vi "P2P SPI Master.vi"() -> ()   [LabVIEW 2015]
uses:
  <vilib>/Platform/TimedLoop/XDataNode/timing_clust.ctl
  <vilib>/Platform/TimedLoop/XDataNode/nitl_modes.ctl
  <vilib>/Platform/TimedLoop/XDataNode/wakeup.ctl
  <vilib>/rvi/Emulation/niFpgaSctlEmulationGetInTimedLoop.vi
  <vilib>/rvi/Emulation/niFpgaEmulationReportErrorSimple.vi
  <vilib>/rvi/Emulation/niFpgaGetClockAttributes.vi
  <vilib>/rvi/Emulation/niFpgaCriticalErrorInLSC.vi
  <vilib>/rvi/Emulation/niFpgaEmulationIsFPGAContextNoSignature.vi
  <vilib>/rvi/errors/niFpgaSetErrorForExecOnDevCompSimple.vi
  <vilib>/rvi/eio/common/nirviEmuReportErrorAndStop.vi
  <vilib>/rvi/DataTransferAndStorage/Container/Common/niFpgaContainerGetUniqueNameForEmu.vi
  <vilib>/rvi/FIFO/Fifo_Resource/nirvififoEmulationSetSize.vi
  <vilib>/rvi/FIFO/Fifo_Resource/nirviFifoEmulationQueueMgr.vi
  <instcachedir>/0/nirviFifoEmulationQueueMgr_E5CAEC123FF24DC58D834DCA3CDAA9B5.lvgen/nirviFifoEmulationQueueMgr_E5CAEC123FF24DC58D834DCA3CDAA9B5_001.vi
  <vilib>/Utility/error.llb/Clear Errors.vi
  <vilib>/rvi/FIFO/Fifo_Resource/nirvififoEmulationCreateLock.vi
  <vilib>/rvi/Emulation/niFpgaProcessEmulError.vi
  <vilib>/rvi/FIFO/Fifo_Resource/nirvififoEmulationObtainLock.vi
  <vilib>/rvi/FIFO/Fifo_Resource/nirvififoEmulationReleaseLock.vi
  <vilib>/rvi/occurrence/nirviWaitOnOccurrenceBase.vi
  <vilib>/rvi/errors/nirviReportUnexpectedCaseInternalError.vi
  <vilib>/rvi/errors/nirviReportUnexpectedCaseInternalError (U32).vi
  <vilib>/rvi/eio/common/nirviEmuTemplateMethod_errors.vi
  <vilib>/Platform/TimedLoop/XDataNode/XDataNode.xnode
  <vilib>/rvi/DataTransferAndStorage/Container/XNode/niFpgaContainer.xnode
  <vilib>/rvi/FIFO/Fifo_Resource/nirvififoEmulationRead.vi
  <vilib>/eio/EIONode/EIONode.xnode
  <vilib>/Platform/TimedLoop/XDataNode/XDNodeRunTimeDep.lvlib
  <vilib>/rvi/FIFO/Fifo_Resource/nirvififoEmulationWrite.vi
panel:
  out "SatePassed":u32
  out "clk":bool
  out "t7":bool
  out "t6":bool
  out "t5":bool
  out "t4":bool
  out "t3":bool
  in  "SimSend":bool
  in  "SimData":u32
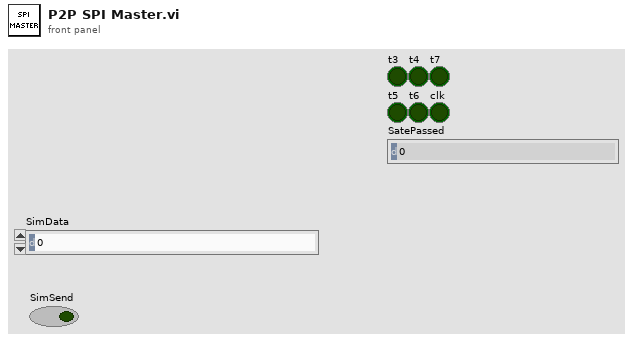
[diagram p1: front panel]
types:
  T1 = typedef "XDNodeRunTimeDep.lvlib/timing_clust.ctl" = cluster{"Expected End [f-1]":u64, "Actual End [f-1]":u64, "Finished Late? [f-1]":bool, "Expected End [i-1]":u64, "Actual End [i-1]":u64, "Finished Late? [i-1]":bool, "Expected Start [i]":u64, "Actual Start [i]":u64, "Expected Start [f]":u64, "Actual Start [f]":u64, "Source Name":string, "Structure Name":string, "Period":i64, "Deadline":i64, "Offset":i64, "Start":i64, "Priority":i32, "Timeout":i32, "Mode":T2, "Wakeup Reason":T3, "Error":errorcluster, "Source Type":string, "Secondary Source Type":string, "Global End Time":u64, "Global Start Time":u64, "Frame Duration":u64, "Iteration Duration":u64, "Assigned CPU":i32, "I/O Scan Engine Mode":u32}
  T2 = typedef "XDNodeRunTimeDep.lvlib/nitl_modes.ctl" = enum32{"No Change", "Process missed periods, maintain original phase", "Discard missed periods, maintain original phase", "Process missed periods, ignore original phase", "Discard missed periods, ignore original phase"}
  T3 = typedef "XDNodeRunTimeDep.lvlib/wakeup.ctl" = enum32{"Normal", "Aborted", "Asynchronous wakeup", "Timing source error", "Timed loop error", "Timeout"}
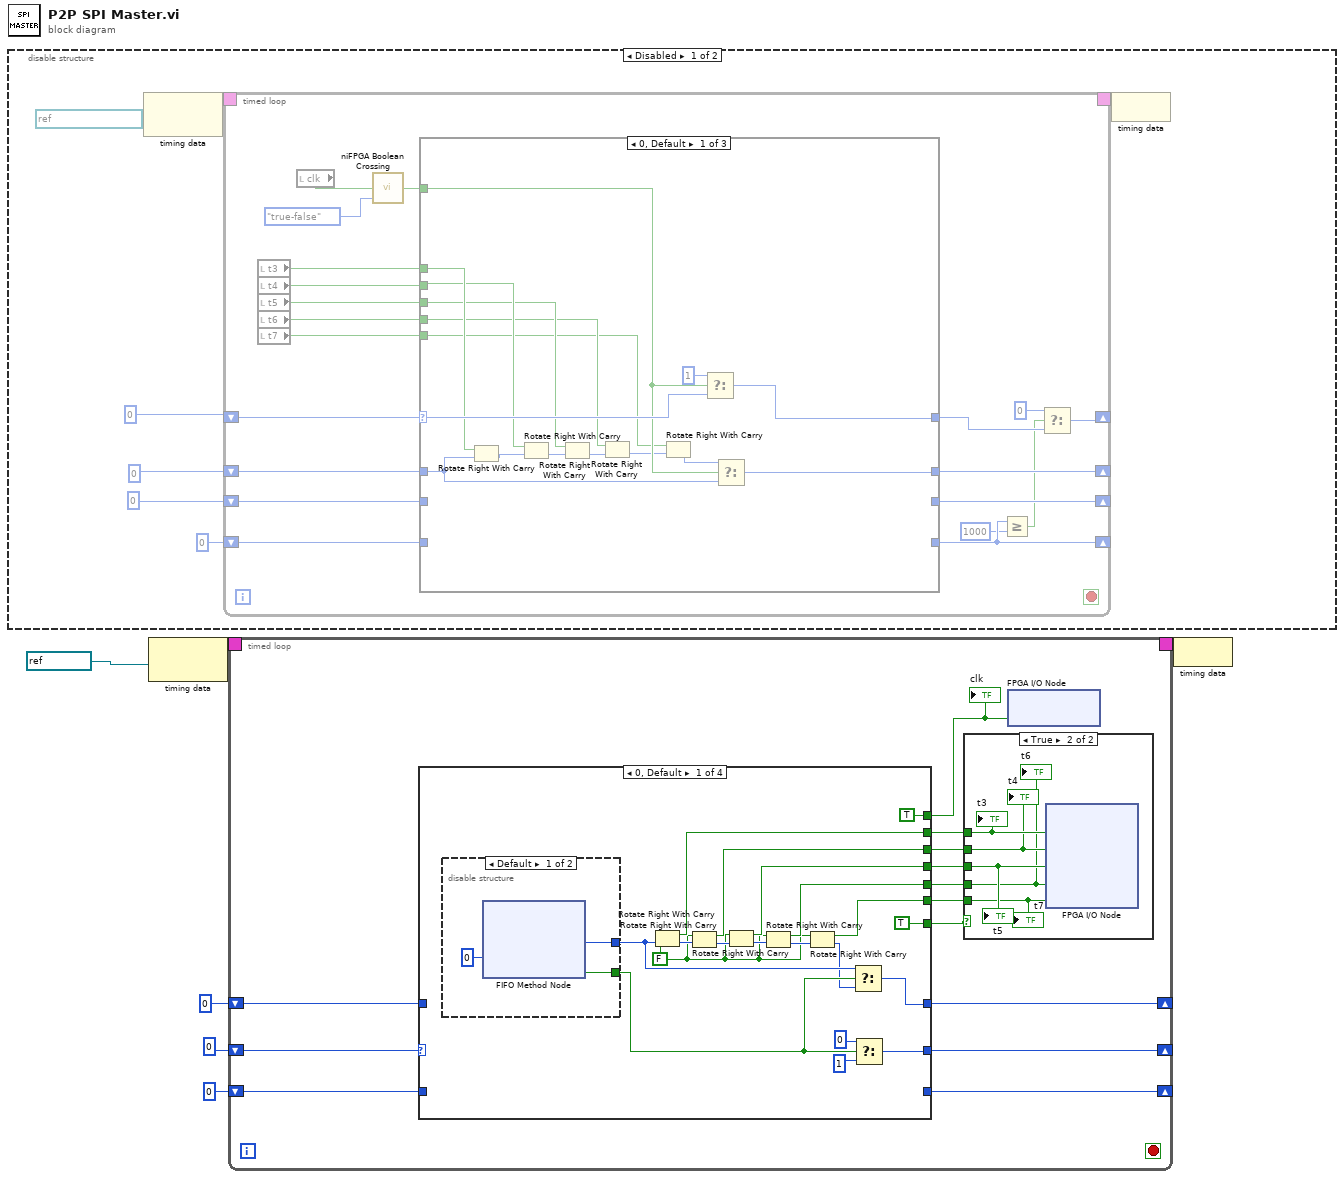
[diagram p0: block diagram]
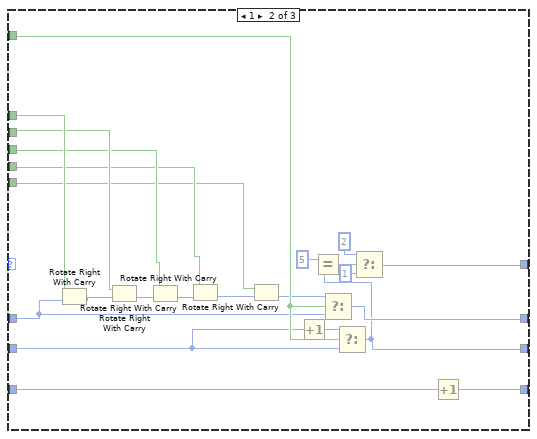
[diagram p2: hidden frame]
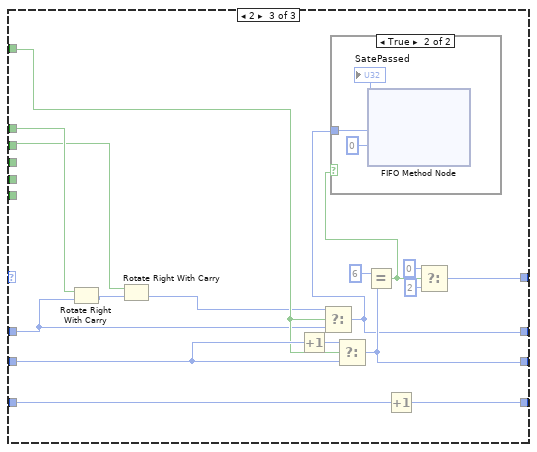
[diagram p3: hidden frame]
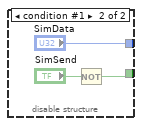
[diagram p7: hidden frame]
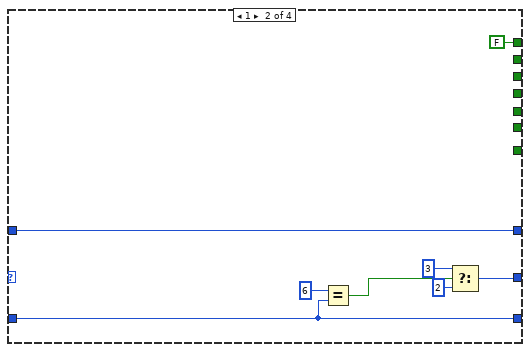
[diagram p8: hidden frame]
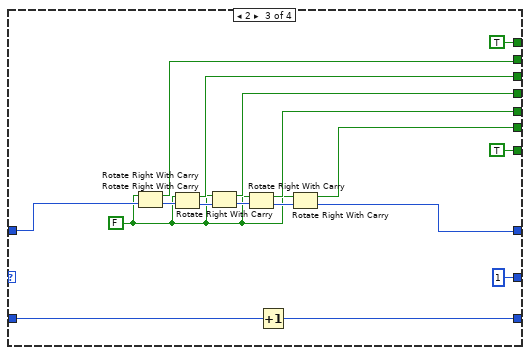
[diagram p9: hidden frame]
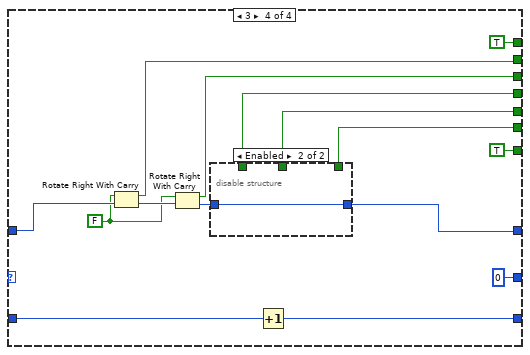
[diagram p10: hidden frame]
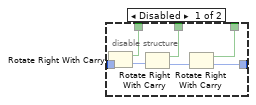
[diagram p11: hidden frame]
diagram:
  n1 = disable-structure shown="Disabled" {
    frame Disabled {
      n2 = node-c288(refnum<k21> "200 MHz Clock" ("Source Name")) -> (w13:T1)
      n3 = timed-loop {
        timing: w13 -> [_]
        timing-out: [_] -> w12
        shift-right: [w16] -> _
        shift-left: u8 0 -> [w33]
        shift-right: [w29] -> _
        shift-left: u32 0 -> [w30]
        shift-right: [w17] -> _
        shift-left: u8 0 -> [w28]
        shift-right: [w26] -> _
        shift-left: 0 -> [w27]
        stop <- _ stop-if-true
        n4 = local read "t3"() -> (w22:bool)
        n5 = local read "t4"() -> (w21:bool)
        n6 = local read "t5"() -> (w20:bool)
        n7 = local read "t6"() -> (w19:bool)
        n8 = local read "t7"() -> (w18:bool)
        n9 = local read "clk"() -> (w23:bool)
        n10 = call <vilib>:"niFPGA Boolean Crossing.vi"("input"=w23, "direction"=enum8{"either", "false-true", "true-false"}."true-false") -> ("crossing"=w32:bool)  [unwired: 7 in]
        n11 = case shown="0, Default" w33 {
          selector: w33 -> [w48 _ _]
          tunnel: w32 -> [w46 w71 w82]
          tunnel: [w49 w68 w87] -> w15
          tunnel: w30 -> [w43 w50 w75]
          tunnel: w22 -> [w44 w56 w76]
          tunnel: [w45 w70 w80] -> w29
          tunnel: w28 -> [_ w67 w86]
          tunnel: [_ w66 w85] -> w17
          tunnel: w21 -> [w41 w55 w74]
          tunnel: w20 -> [w40 w54 _]
          tunnel: w19 -> [w39 w53 _]
          tunnel: w18 -> [w38 w52 _]
          tunnel: [_ w61 w78] -> w26
          tunnel: w27 -> [_ w62 w79]
          frame 0, Default {
            n12 = Rotate Right With Carry(2:w43, 3:w44) -> (0:w37:u32)  [unwired: 1 out]
            n13 = Rotate Right With Carry(2:w37, 3:w41) -> (0:w36:u32)  [unwired: 1 out]
            n14 = Rotate Right With Carry(2:w36, 3:w40) -> (0:w35:u32)  [unwired: 1 out]
            n15 = Rotate Right With Carry(2:w35, 3:w39) -> (0:w34:u32)  [unwired: 1 out]
            n16 = Rotate Right With Carry(2:w34, 3:w38) -> (0:w42:u32)  [unwired: 1 out]
            n17 = Select(t=u8 1, s=w46, f=w48) -> (s? t:f=w49:u8)
            n18 = Select(t=w42, s=w46, f=w43) -> (s? t:f=w45:u32)
          }
          frame 1 {
            n19 = Rotate Right With Carry(2:w50, 3:w56) -> (0:w60:u32)  [unwired: 1 out]
            n20 = Rotate Right With Carry(2:w60, 3:w55) -> (0:w59:u32)  [unwired: 1 out]
            n21 = Rotate Right With Carry(2:w59, 3:w54) -> (0:w58:u32)  [unwired: 1 out]
            n22 = Rotate Right With Carry(2:w58, 3:w53) -> (0:w57:u32)  [unwired: 1 out]
            n23 = Rotate Right With Carry(2:w57, 3:w52) -> (0:w51:u32)  [unwired: 1 out]
            n24 = Increment(x=w67) -> (x+1=w72:u8)
            n25 = Select(t=w51, s=w71, f=w50) -> (s? t:f=w70:u32)
            n26 = Select(t=w72, s=w71, f=w67) -> (s? t:f=w66:u8)
            n27 = Equal?(x=u8 5, y=w66) -> (x = y?=w65:bool)
            n28 = Select(t=u8 2, s=w65, f=u8 1) -> (s? t:f=w68:u8)
            n29 = Increment(x=w62) -> (x+1=w61:i32)
          }
          frame 2 {
            n30 = Rotate Right With Carry(2:w75, 3:w76) -> (0:w77:u32)  [unwired: 1 out]
            n31 = Rotate Right With Carry(2:w77, 3:w74) -> (0:w73:u32)  [unwired: 1 out]
            n32 = Increment(x=w86) -> (x+1=w89:u8)
            n33 = Select(t=w73, s=w82, f=w75) -> (s? t:f=w80:u32)
            n34 = Select(t=w89, s=w82, f=w86) -> (s? t:f=w85:u8)
            n35 = Equal?(x=u8 6, y=w85) -> (x = y?=w81:bool)
            n36 = case shown="True" w81 {
              tunnel: w80 -> [_ w90]
              frame False {
              }
              frame True {
                n37 = xnode ("FIFO Method Node")("Element"=w90, "Timeout"=0) -> ()  [unwired: 1 in, 2 out]
                "SatePassed" <- w90
              }
            }
            n38 = Increment(x=w79) -> (x+1=w78:i32)
            n39 = Select(t=u8 0, s=w81, f=u8 2) -> (s? t:f=w87:u8)
          }
        }
        n40 = Greater Or Equal?(x=w26, y=1000) -> (x >= y?=w14:bool)
        n41 = Select(t=u8 0, s=w14, f=w15) -> (s? t:f=w16:u8)
      }
      n42 = node-c288(w12) -> ()
    }
    frame Enabled {
    }
  }
  n43 = node-c288(refnum<k21> "80MHz" ("Source Name")) -> (w6:T1)
  n44 = timed-loop {
    timing: w6 -> [_]
    timing-out: [_] -> w5
    shift-right: [w109] -> _
    shift-left: 0 -> [w110]
    shift-right: [w108] -> _
    shift-left: u32 0 ("Element") -> [w100]
    shift-right: [w98] -> _
    shift-left: 0 -> [w99]
    stop <- _ stop-if-true
    n45 = case shown="0, Default" w110 {
      tunnel: [TRUE ("Timed Out?") FALSE ("Timed Out?") TRUE ("Timed Out?") TRUE ("Timed Out?")] -> w102
      tunnel: [w132 w142 1 0] -> w109
      tunnel: [w125 w147 w155 w172] -> w108
      tunnel: [w123 _ w160 w177] -> w107
      tunnel: [w122 _ w159 w176] -> w106
      tunnel: [w121 _ w158 w175] -> w105
      tunnel: [w120 _ w157 w174] -> w104
      tunnel: [w119 _ w156 w173] -> w103
      tunnel: [TRUE _ TRUE TRUE] -> w101
      tunnel: w100 -> [_ w147 w161 w178]
      tunnel: w99 -> [_ w145 w151 w168]
      tunnel: [_ w145 w150 w167] -> w98
      frame 0, Default {
        w116 = FALSE
        n46 = disable-structure shown="Default" {
          disable-tunnel: [w136 w138] -> w127
          disable-tunnel: [w135 "SimData"] -> w126
          frame condition #0 (active) {
            n47 = xnode ("FIFO Method Node")("Timeout"=0) -> ("Element"=w135:u32, "Timed Out?"=w136:bool)  [unwired: 1 in, 1 out]
          }
          frame condition #1 {
            n48 = Not(x="SimSend") -> (.not. x?=w138:bool)
          }
        }
        n49 = Rotate Right With Carry(2:w126, 3:w116) -> (0:w131:u32, 1:w123:bool)
        n50 = Rotate Right With Carry(2:w131, 3:w116) -> (0:w130:u32, 1:w122:bool)
        n51 = Rotate Right With Carry(2:w130, 3:w116) -> (0:w129:u32, 1:w121:bool)
        n52 = Rotate Right With Carry(2:w129, 3:w116) -> (0:w128:u32, 1:w120:bool)
        n53 = Rotate Right With Carry(2:w128, 3:w116) -> (0:w124:u32, 1:w119:bool)
        n54 = Select(t=w126, s=w127, f=w124) -> (s? t:f=w125:u32)
        n55 = Select(t=0, s=w127, f=1) -> (s? t:f=w132:i32)
      }
      frame 1 {
        n56 = Equal?(x=6, y=w145) -> (x = y?=w143:bool)
        n57 = Select(t=3, s=w143, f=2) -> (s? t:f=w142:i32)
      }
      frame 2 {
        w149 = FALSE
        n58 = Rotate Right With Carry(2:w161, 3:w149) -> (0:w165:u32, 1:w160:bool)
        n59 = Rotate Right With Carry(2:w165, 3:w149) -> (0:w164:u32, 1:w159:bool)
        n60 = Rotate Right With Carry(2:w164, 3:w149) -> (0:w163:u32, 1:w158:bool)
        n61 = Rotate Right With Carry(2:w163, 3:w149) -> (0:w162:u32, 1:w157:bool)
        n62 = Increment(x=w151) -> (x+1=w150:i32)
        n63 = Rotate Right With Carry(2:w162, 3:w149) -> (0:w155:u32, 1:w156:bool)
      }
      frame 3 {
        w166 = FALSE
        n64 = Rotate Right With Carry(2:w178, 3:w166) -> (0:w180:u32, 1:w177:bool)
        n65 = Rotate Right With Carry(2:w180, 3:w166) -> (0:w179:u32, 1:w176:bool)
        n66 = disable-structure shown="Enabled" {
          disable-tunnel: w179 -> [w187 w188]
          disable-tunnel: [w184 _] -> w175
          disable-tunnel: [w183 _] -> w174
          disable-tunnel: [w182 _] -> w173
          disable-tunnel: [w181 w188] -> w172
          frame Disabled {
            n67 = Rotate Right With Carry(2:w187) -> (0:w186:u32, 1:w184:bool)  [unwired: 1 in]
            n68 = Rotate Right With Carry(2:w186) -> (0:w185:u32, 1:w183:bool)  [unwired: 1 in]
            n69 = Rotate Right With Carry(2:w185) -> (0:w181:u32, 1:w182:bool)  [unwired: 1 in]
          }
          frame Enabled {
          }
        }
        n70 = Increment(x=w168) -> (x+1=w167:i32)
      }
    }
    "clk" <- w102
    n71 = case shown="True" w101 {
      tunnel: w107 -> [_ w115]
      tunnel: w106 -> [_ w114]
      tunnel: w105 -> [_ w113]
      tunnel: w104 -> [_ w112]
      tunnel: w103 -> [_ w111]
      frame False {
      }
      frame True {
        n72 = xnode "FPGA I/O Node"("PXI_Trig3"=w115, "PXI_Trig4"=w114, "PXI_Trig5"=w113, "PXI_Trig6"=w112, "PXI_Trig7"=w111) -> ()  [unwired: 5 in, 5 out]
        "t3" <- w115
        "t4" <- w114
        "t5" <- w113
        "t6" <- w112
        "t7" <- w111
      }
    }
    n73 = xnode "FPGA I/O Node"("PXI_Trig2"=w102) -> ()  [unwired: 1 in, 1 out]
  }
  n74 = node-c288(w5) -> ()
